vi "Close.vi"(11 "Handle":i32) -> (2 "Return":i32, 3 "Handle out":i32)   [LabVIEW 2022 SP3]
doc: "BOOL H11890API __stdcall H11890Close(HANDLE hDeviceHandle);"
uses:
  EXE/data/H11890api.dll
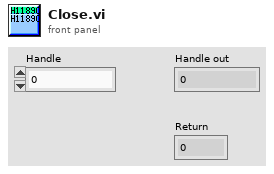
[diagram p1: front panel]
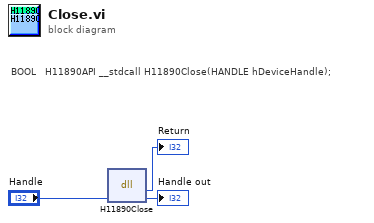
[diagram p0: block diagram]
diagram:
  # "BOOL\t\t\tH11890API __stdcall H11890Close(HANDLE hDeviceHandle);"
  n1 = dll-call lib="C:/Users/Public/OneDrive/Desktop/PMT program/SampleCodeLabView/EXE/data/H11890api.dll" fn="H11890Close"("Handle"="Handle") -> ("Return"=→"Return":i32, "Handle"=→"Handle out":i32)  [unwired: 3 in, 2 out]
